vi "Target Groups.vi"(8 "error in (no error)":errorcluster, 11 "Node in":refnum<class "Node.lvclass">) -> (0 "error out":errorcluster, 2 "Target Groups":string[](array[string]), 3 "Node out":refnum<class "Node.lvclass">)   [LabVIEW 2020, in "VolatusConfig.lvlib" / "Node.lvclass"]
uses:
  Node.lvclass
  Node.lvclass/Node.ctl
  VolatusConfigElement/VolatusConfigElement.lvclass
  lv-cdm/CDM-Config/Config Element/Config Element.lvclass
  C:/dev/lv20CE/relink/lv-volatus/VolatusConfig/VolatusConfigElement/VolatusConfigElement.lvclass
  C:/dev/lv20CE/relink/lv-volatus/VolatusConfig/Node/Node.lvclass
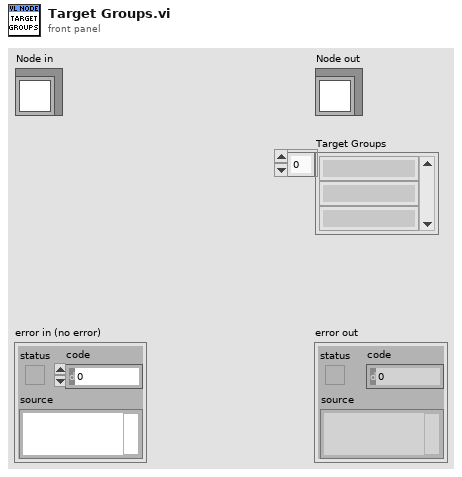
[diagram p1: front panel]
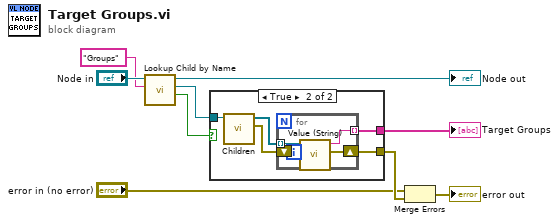
[diagram p0: block diagram]
diagram:
  n1 = call "Lookup Child by Name.vi"("Child Name"="Groups", "VolatusConfigElement in"="Node in") -> ("Found"=w4:bool, "Child"=w6:refnum<class "Config Element.lvclass">, "VolatusConfigElement out"=→"Node out":refnum<class "Node.lvclass">)  [unwired: 6 in, 1 out]
  n2 = case shown="True" w4 {
    tunnel: w6 -> [_ w14]
    tunnel: [_ w11] -> w5
    tunnel: [_ w10] -> w3
    frame False {
      # "Groups are optional"
    }
    frame True {
      n3 = call "Children.vi"("Config Element in"=w14) -> ("error out"=w12:errorcluster, "Elements"=w13:refnum<class "Config Element.lvclass">[])  [unwired: 9 in]
      n4 = for {
        tunnel: w13 -> [w18] mode=indexing
        shift-right: [w16] -> w10
        shift-left: w12 -> [w17]
        tunnel: [w15] -> w11 mode=indexing
        n5 = call "Value (String).vi"("error in (no error)"=w17, "Config Element in"=w18) -> ("error out"=w16:errorcluster, "String Value"=w15:string)  [unwired: 8 in]
      }
    }
  }
  "Target Groups" <- w5
  n6 = Merge Errors("error in (no error)", w3) -> (→"error out":errorcluster)
